vi "Model 3566-Request.vi"(8 "error in":errorcluster, 10 "Command":string, 11 "Model 3566 Setting In":T1) -> (0 "error out":errorcluster, 2 "Respond":string, 3 "Model 3566 Setting Out":T1)   [LabVIEW 2018]
uses:
  Data Def/Model 3566-Setting.ctl
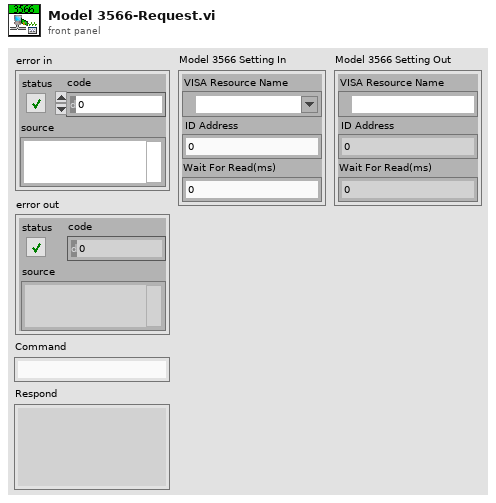
[diagram p1: front panel]
types:
  T1 = typedef "Model 3566-Setting.ctl" = cluster{"VISA Resource Name":refnum<visa-resource-name>, "ID Address":u8, "Wait For Read(ms)":u32}
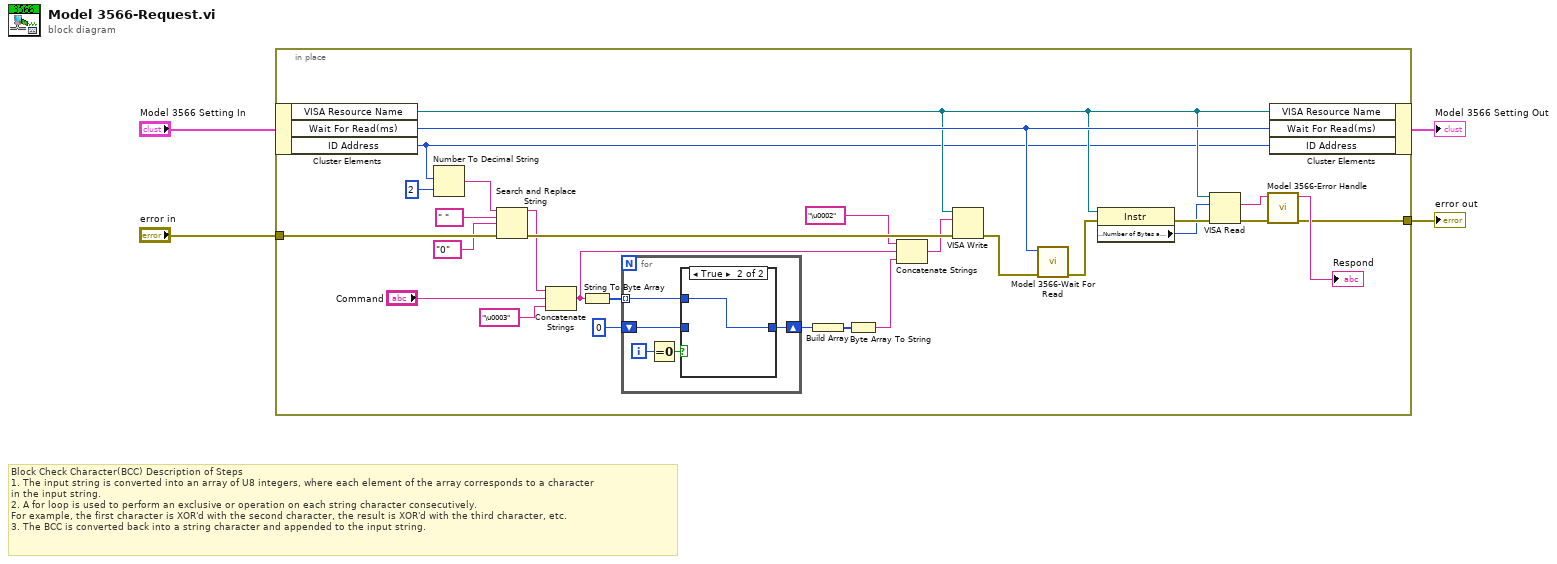
[diagram p0: block diagram]
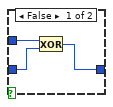
[diagram p2: hidden frame]
diagram:
  # "Block Check Character(BCC) Description of Steps\n1. The input string is converted into an array of U8 integers, where each element of the array corresponds to a character\nin the input string.\n2. A for loop is used to perform an exclusive or operation on each string character consecutively.  \nFor example, the first character is XOR'd with the second character, the result is XOR'd with the third character, etc.\n3. The BCC is converted back into a string character and appended to the input string."
  n1 = in-place {
    in-place-border: "error in" -> [w20]
    in-place-border: [w24] -> w1
    n2 = in-place-cluster #1("Model 3566 Setting In") -> ("VISA Resource Name"=w23:refnum<visa-resource-name>, "Wait For Read(ms)"=w25:u32, "ID Address"=w22:u8)
    n3 = Number To Decimal String(number=w22, width (-)=i16 2) -> (decimal integer string=w18:string)
    n4 = Search and Replace String(input string=w18, search string=" ", replace string="0" ("replace string (\"\")"), error in=w20) -> (result string=w15:string, error out=w19:errorcluster)  [unwired: 4 in, 2 out]
    n5 = Concatenate Strings(w15, "Command", "\u0003" ("replace string (\"\")")) -> (w10:string)
    n6 = String To Byte Array(string=w10) -> (unsigned byte array=w12:u8[])
    n7 = for {
      tunnel: w12 -> [w35] mode=indexing
      shift-right: [w33] -> w7
      shift-left: u8 0 -> [w34]
      i -> [w37]
      n8 = Equal To 0?(x=w37) -> (x = 0?=w36:bool)
      n9 = case shown="True" w36 {
        tunnel: w35 -> [w40 w41]
        tunnel: w34 -> [w39 _]
        tunnel: [w38 w41] -> w33
        frame False {
          n10 = Exclusive Or(1:w39, 2:w40) -> (0:w38:u8)
        }
        frame True {
        }
      }
    }
    n11 = Build Array(w7) -> (w6:u8[])
    n12 = Byte Array To String(unsigned byte array=w6) -> (string=w5:string)
    n13 = Concatenate Strings("\u0002" ("replace string (\"\")"), w10, w5) -> (w8:string)
    n14 = VISA Write(VISA resource name=w23, write buffer=w8, error in (no error)=w19) -> (error out=w32:errorcluster)  [unwired: 2 out]
    n15 = call "Model 3566-Wait For Read.vi"("error in"=w32, "Wait For Read(ms)"=w25) -> ("error out"=w31:errorcluster)  [unwired: 9 in]
    n16 = property class="Instr"(reference=w23, error in=w31) -> (error out=w30:errorcluster, "Serial Settings:Number of Bytes at Serial Port"=w29:u32)  [unwired: 1 out]
    n17 = VISA Read(VISA resource name=w23, byte count=w29, error in (no error)=w30) -> (read buffer=w27:string, error out=w28:errorcluster)  [unwired: 2 out]
    n18 = call "Model 3566-Error Handle.vi"("error in"=w28, "Respond In"=w27) -> ("error out"=w24:errorcluster, "Respond Out"=→"Respond":string)  [unwired: 8 in]
    n19 = in-place-cluster #1("VISA Resource Name"=w23, "Wait For Read(ms)"=w25, "ID Address"=w22) -> (→"Model 3566 Setting Out":T1)
  }
  "error out" <- w1
